vi "Set DDS Pinlv.vi"(8 "error in (no error)":errorcluster, 10 "pinlv":u32, 11 "channel_index":u8) -> (0 "error out":errorcluster)   [LabVIEW 2021, in "vmmsolib.lvlib"]
doc: "DLL_API void WINAPI SetDDSPinlv(unsigned char channel_index, unsigned int pinlv);"
uses:
  vmmsolib.lvlib
  vmmso.dll
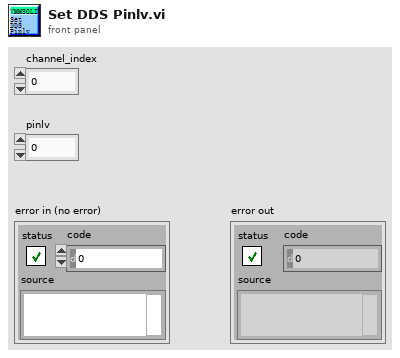
[diagram p1: front panel]
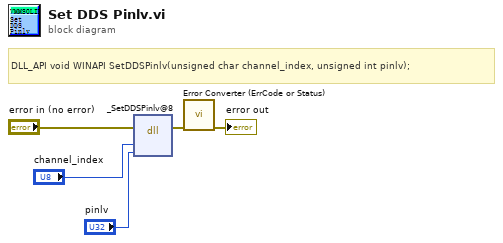
[diagram p0: block diagram]
diagram:
  # "DLL_API void WINAPI SetDDSPinlv(unsigned char channel_index, unsigned int pinlv);"
  n1 = dll-call lib="D:/VmMsoSDK/demo-Labview/2021/vmmsolib/vmmso.*" fn="_SetDDSPinlv@8"(error in="error in (no error)", "channel_index"="channel_index", "pinlv"="pinlv") -> (error out=w2:errorcluster)  [unwired: 5 in, 1 out]
  n2 = call "Error Converter (ErrCode or Status).vi"("error in (no error)"=w2) -> ("error out"=→"error out":errorcluster)  [unwired: 10 in]
